vi "NI VeriStand - Set Item Property.vi"   [LabVIEW 2020, in "Custom Device API.lvlib"]
doc: "Sets a <B>Property Name</B> and <B>Value</B> for an item property and saves this information in the system definition file. If the <B>Property Name</B> you specify already exists, this VI overwrites the property. Wire data to the <B>Value</B> input to determine the polymorphic instance to use or manually select the instance."
uses:
  <vilib>/NI VeriStand/Custom Device API/Custom Device API.lvlib
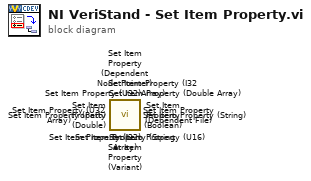
[diagram p0: block diagram]
diagram:
  n1 = call <vilib>:"Set Item Property (String Array).vi"() -> ()  [unwired: 9 in, 3 out]
  n2 = call <vilib>:"Set Item Property (I32 Array).vi"() -> ()  [unwired: 9 in, 3 out]
  n3 = call <vilib>:"Set Item Property (U32 Array).vi"() -> ()  [unwired: 9 in, 3 out]
  n4 = call <vilib>:"Set Item Property (Dependent File).vi"() -> ()  [unwired: 9 in, 3 out]
  n5 = call <vilib>:"Set Item Property (U32).vi"() -> ()  [unwired: 9 in, 3 out]
  n6 = call <vilib>:"Set Item Property (Dependent Node Pointer).vi"() -> ()  [unwired: 9 in, 3 out]
  n7 = call <vilib>:"Set Item Property (Variant).vi"() -> ()  [unwired: 9 in, 3 out]
  n8 = call <vilib>:"Set Item Property (U16).vi"() -> ()  [unwired: 9 in, 3 out]
  n9 = call <vilib>:"Set Item Property (String).vi"() -> ()  [unwired: 9 in, 3 out]
  n10 = call <vilib>:"Set Item Property (Path).vi"() -> ()  [unwired: 9 in, 3 out]
  n11 = call <vilib>:"Set Item Property (I32).vi"() -> ()  [unwired: 9 in, 3 out]
  n12 = call <vilib>:"Set Item Property (Double).vi"() -> ()  [unwired: 9 in, 3 out]
  n13 = call <vilib>:"Set Item Property (Double Array).vi"() -> ()  [unwired: 9 in, 3 out]
  n14 = call <vilib>:"Set Item Property (Boolean).vi"() -> ()  [unwired: 9 in, 3 out]
